vi "TryUpdateDisplacementSample.vi"   [LabVIEW 2016]
uses:
  TelemetryDataTypes.ctl
  TelemetryUpdateModes.ctl
  TelemetryFields.ctl
  <vilib>/rvi/Emulation/niFpgaEmulationIsFPGAContextNoSignature.vi
  <vilib>/rvi/Emulation/niFpgaSctlEmulationGetInTimedLoop.vi
  <vilib>/rvi/errors/niFpgaSetErrorForExecOnDevCompSimple.vi
  <vilib>/rvi/eio/common/nirviEmuReportErrorAndStop.vi
  <vilib>/rvi/DataTransferAndStorage/Container/Common/niFpgaContainerGetUniqueNameForEmu.vi
  <vilib>/rvi/FIFO/Fifo_Resource/nirvififoEmulationSetSize.vi
  <vilib>/rvi/FIFO/Fifo_Resource/nirviFifoEmulationQueueMgr.vi
  <instcachedir>/0/nirviFifoEmulationQueueMgr_E5CAEC123FF24DC58D834DCA3CDAA9B5.lvgen/nirviFifoEmulationQueueMgr_E5CAEC123FF24DC58D834DCA3CDAA9B5_028.vi
  <vilib>/Utility/error.llb/Clear Errors.vi
  <vilib>/rvi/FIFO/Fifo_Resource/nirvififoEmulationCreateLock.vi
  <vilib>/rvi/Emulation/niFpgaProcessEmulError.vi
  <vilib>/rvi/FIFO/Fifo_Resource/nirvififoEmulationObtainLock.vi
  <vilib>/rvi/FIFO/Fifo_Resource/nirvififoEmulationReleaseLock.vi
  <vilib>/rvi/occurrence/nirviWaitOnOccurrenceBase.vi
  <vilib>/rvi/errors/nirviReportUnexpectedCaseInternalError.vi
  <vilib>/rvi/errors/nirviReportUnexpectedCaseInternalError (U32).vi
  <instcachedir>/0/nirviFifoEmulationQueueMgr_E5CAEC123FF24DC58D834DCA3CDAA9B5.lvgen/nirviFifoEmulationQueueMgr_E5CAEC123FF24DC58D834DCA3CDAA9B5_030.vi
  <vilib>/rvi/FIFO/Fifo_Resource/nirvififoEmulationDetermineInputValidOut.vi
  <instcachedir>/0/nirviFifoEmulationQueueMgr_E5CAEC123FF24DC58D834DCA3CDAA9B5.lvgen/nirviFifoEmulationQueueMgr_E5CAEC123FF24DC58D834DCA3CDAA9B5_031.vi
  <vilib>/rvi/Emulation/niFpgaGetClockAttributes.vi
  <vilib>/rvi/Emulation/niFpgaEmulationReportErrorSimple.vi
  <vilib>/rvi/Memory/Memory_Emulation/niFpgaMemoryEmulationCacheClearOnFirstRun.vi
  <vilib>/rvi/Memory/Memory_Emulation/nirvimemoryEmulationManagerCache_MakeExclusive.vi
  <vilib>/rvi/Memory/Memory_Emulation/niFpgaMemoryEmulationValidateCache.vi
  <vilib>/rvi/Memory/Memory_Emulation/nirvimemoryEmulationManagerCache_InsertValue.vi
  <vilib>/rvi/Memory/Memory_Emulation/nirvimemoryEmulationManagerCache_ReleaseExclusive.vi
  <vilib>/rvi/Memory/Memory_Emulation/nirvimemoryEmulationManagerCache_GetValue.vi
  <vilib>/rvi/Memory/Memory_Emulation/nirvimemoryEmulationManagerCache_SetValue.vi
  <vilib>/rvi/Emulation/niFpgaCriticalErrorInLSC.vi
  <instcachedir>/0/nirviFifoEmulationQueueMgr_E5CAEC123FF24DC58D834DCA3CDAA9B5.lvgen/nirviFifoEmulationQueueMgr_E5CAEC123FF24DC58D834DCA3CDAA9B5_004.vi
  <vilib>/rvi/DataTransferAndStorage/Container/XNode/niFpgaContainer.xnode
  <vilib>/rvi/FIFO/Fifo_Resource/nirvififoEmulationRead.vi
  <vilib>/rvi/FIFO/Fifo_Resource/nirvififoEmulationWrite.vi
  <vilib>/rvi/DataTransferAndStorage/Register/Emulation/niFpgaRegisterEmulation.vi
  Displacement/DisplacementErrorCodes.ctl
types:
  T1 = cluster{"Timestamp":u64, "TxBytes":u64, "RxBytes":u64, "TxFrames":u64, "RxFrames":u64, "Sensor1Raw":i32, "Sensor2Raw":i32, "Sensor3Raw":i32, "Sensor4Raw":i32, "Sensor5Raw":i32, "Sensor6Raw":i32, "Sensor7Raw":i32, "Sensor8Raw":i32, "Sensor1Eng":sgl, "Sensor2Eng":sgl, "Sensor3Eng":sgl, "Sensor4Eng":sgl, "Sensor5Eng":sgl, "Sensor6Eng":sgl, "Sensor7Eng":sgl, "Sensor8Eng":sgl, "PositionX":sgl, "PositionY":sgl, "PositionZ":sgl, "RotationX":sgl, "RotationY":sgl, "RotationZ":sgl}
  T2 = typedef "TelemetryFields.ctl" = enum16{"None", "InclinometerTxBytes", "InclinometerRxBytes", "InclinometerTxFrames", "InclinometerRxFrames", "InclinometerErrorTimestamp", "InclinometerErrorCode", "InclinometerSampleTimestamp", "InclinometerRawAngle", "InclinometerZenithAngle", "DisplacementTxBytes", "DisplacementRxBytes", "DisplacementTxFrames", "DisplacementRxFrames", "DisplacementErrorTimestamp", "DisplacementErrorCode", "DisplacementSampleTimestamp", "DisplacementRaw1", "DisplacementRaw2", "DisplacementRaw3", "DisplacementRaw4", "DisplacementRaw5", "DisplacementRaw6", "DisplacementRaw7", "DisplacementRaw8", "DisplacementEng1", "DisplacementEng2", "DisplacementEng3", "DisplacementEng4", "DisplacementEng5", "DisplacementEng6", "DisplacementEng7", "DisplacementEng8", "DisplacementPositionX", "DisplacementPositionY", "DisplacementPositionZ", "DisplacementRotationX", "DisplacementRotationY", "DisplacementRotationZ", "AccelerometerSampleCount", "AccelerometerTimestamp", "AccelerometerRaw1", "AccelerometerRaw2", "AccelerometerRaw3", "AccelerometerRaw4", "AccelerometerRaw5", "AccelerometerRaw6", "AccelerometerRaw7", "AccelerometerRaw8", "AccelerometerEng1", "AccelerometerEng2", "AccelerometerEng3", "AccelerometerEng4", "AccelerometerEng5", "AccelerometerEng6", "AccelerometerEng7", "AccelerometerEng8", "AngularAccelerationX", "AngularAccelerationY", "AngularAccelerationZ"}
  T3 = typedef "TelemetryUpdateModes.ctl" = enum8{"=", "+", "-", "|"}
  T4 = typedef "TelemetryDataTypes.ctl" = enum8{"U8", "U16", "U32", "U64", "I8", "I16", "I32", "I64", "SGL"}
  T5 = typedef "DisplacementErrorCodes.ctl" = enum16{"None", "ResponseUnknownError", "ResponseInvalidError", "ResponseTimeoutError", "SensorIndicatesInvalidCommandError", "SensorIndicatesCommunicationTimeoutError", "SensorIndicatesDataLengthError", "SensorIndicatesNumberOfParametersError", "SensorIndicatesParameterError", "SensorIndicatesCommunicationError", "SensorIndicatesIDNumberError", "SensorIndicatesExpansionLineError", "SensorIndicatesWriteControlError"}
  T6 = typedef "TelemetryUpdateData.ctl" = cluster{"DataType":T4, "Mode":T3, "Field":T2, "Data":u64}
  T7 = typedef "TelemetryUpdateDataSGL.ctl" = cluster{"Mode":T3, "Field":T2, "Data":sgl}
diagram:
  n1 = xnode ("FIFO Method Node")("Timeout"=0) -> ("Element"=w1:T1, "Timed Out?"=w2:bool)  [unwired: 1 in, 1 out]
  n2 = case shown="False" w2 {
    tunnel: w1 -> [w4 _]
    frame False {
      n3 = flat-sequence {
        tunnel: w4 -> [w7]
        tunnel: w4 -> [w13]
        tunnel: w4 -> [w21]
        tunnel: w4 -> [w29]
        tunnel: w4 -> [w37]
        tunnel: w4 -> [w46]
        tunnel: w4 -> [w54]
        tunnel: w4 -> [w62]
        tunnel: w4 -> [w70]
        tunnel: w4 -> [w78]
        tunnel: w4 -> [w86]
        tunnel: w4 -> [w94]
        tunnel: w4 -> [w102]
        tunnel: w4 -> [w110]
        tunnel: w4 -> [w116]
        tunnel: w4 -> [w123]
        tunnel: w4 -> [w130]
        tunnel: w4 -> [w137]
        tunnel: w4 -> [w144]
        tunnel: w4 -> [w151]
        tunnel: w4 -> [w158]
        tunnel: w4 -> [w165]
        tunnel: w4 -> [w172]
        tunnel: w4 -> [w179]
        tunnel: w4 -> [w186]
        tunnel: w4 -> [w193]
        tunnel: w4 -> [w200]
        frame #0 {
          n4 = Unbundle By Name(w7) -> ("Timestamp"=w6:u64)
          n5 = call "GetTelemetryUpdateDataConstant.vi"() -> ("TelemetryUpdateData"=w8:T6)  [unwired: 11 in]
          n6 = Bundle By Name(cluster=w8, "DataType"=TelemetryDataTypes."U64", "Mode"=TelemetryUpdateModes."=", "Field"=TelemetryFields."DisplacementSampleTimestamp" ("TelemetryFields"), "Data"=w6) -> (w11:T6)
          n7 = xnode ("FIFO Method Node")("Element"=w11, "Timeout"=-1) -> ()  [unwired: 1 in, 2 out]
        }
        frame #1 {
          n8 = Unbundle By Name(w13) -> ("TxBytes"=w20:u64)
          n9 = call "GetTelemetryUpdateDataConstant.vi"() -> ("TelemetryUpdateData"=w19:T6)  [unwired: 11 in]
          n10 = Bundle By Name(cluster=w19, "DataType"=TelemetryDataTypes."U64", "Mode"=TelemetryUpdateModes."=", "Field"=TelemetryFields."DisplacementTxBytes", "Data"=w20) -> (w15:T6)
          n11 = xnode ("FIFO Method Node")("Element"=w15, "Timeout"=-1) -> ()  [unwired: 1 in, 2 out]
        }
        frame #2 {
          n12 = Unbundle By Name(w21) -> ("RxBytes"=w22:u64)
          n13 = call "GetTelemetryUpdateDataConstant.vi"() -> ("TelemetryUpdateData"=w23:T6)  [unwired: 11 in]
          n14 = Bundle By Name(cluster=w23, "DataType"=TelemetryDataTypes."U64", "Mode"=TelemetryUpdateModes."=", "Field"=TelemetryFields."DisplacementRxBytes", "Data"=w22) -> (w27:T6)
          n15 = xnode ("FIFO Method Node")("Element"=w27, "Timeout"=-1) -> ()  [unwired: 1 in, 2 out]
        }
        frame #3 {
          n16 = Unbundle By Name(w29) -> ("TxFrames"=w36:u64)
          n17 = call "GetTelemetryUpdateDataConstant.vi"() -> ("TelemetryUpdateData"=w35:T6)  [unwired: 11 in]
          n18 = Bundle By Name(cluster=w35, "DataType"=TelemetryDataTypes."U64", "Mode"=TelemetryUpdateModes."=", "Field"=TelemetryFields."DisplacementTxFrames", "Data"=w36) -> (w31:T6)
          n19 = xnode ("FIFO Method Node")("Element"=w31, "Timeout"=-1) -> ()  [unwired: 1 in, 2 out]
        }
        frame #4 {
          n20 = Unbundle By Name(w37) -> ("RxFrames"=w38:u64)
          n21 = call "GetTelemetryUpdateDataConstant.vi"() -> ("TelemetryUpdateData"=w39:T6)  [unwired: 11 in]
          n22 = Bundle By Name(cluster=w39, "DataType"=TelemetryDataTypes."U64", "Mode"=TelemetryUpdateModes."=", "Field"=TelemetryFields."DisplacementRxFrames", "Data"=w38) -> (w43:T6)
          n23 = xnode ("FIFO Method Node")("Element"=w43, "Timeout"=-1) -> ()  [unwired: 1 in, 2 out]
        }
        frame #5 {
          n24 = Unbundle By Name(w46) -> ("Sensor1Raw"=w52:i32)
          n25 = call "GetTelemetryUpdateDataConstant.vi"() -> ("TelemetryUpdateData"=w51:T6)  [unwired: 11 in]
          n26 = Bundle By Name(cluster=w51, "DataType"=TelemetryDataTypes."I32", "Mode"=TelemetryUpdateModes."=", "Field"=TelemetryFields."DisplacementRaw1" ("TelemetryFields"), "Data"=w52) -> (w48:T6)
          n27 = xnode ("FIFO Method Node")("Element"=w48, "Timeout"=-1) -> ()  [unwired: 1 in, 2 out]
        }
        frame #6 {
          n28 = Unbundle By Name(w54) -> ("Sensor2Raw"=w55:i32)
          n29 = call "GetTelemetryUpdateDataConstant.vi"() -> ("TelemetryUpdateData"=w56:T6)  [unwired: 11 in]
          n30 = Bundle By Name(cluster=w56, "DataType"=TelemetryDataTypes."I32", "Mode"=TelemetryUpdateModes."=", "Field"=TelemetryFields."DisplacementRaw2" ("TelemetryFields"), "Data"=w55) -> (w59:T6)
          n31 = xnode ("FIFO Method Node")("Element"=w59, "Timeout"=-1) -> ()  [unwired: 1 in, 2 out]
        }
        frame #7 {
          n32 = Unbundle By Name(w62) -> ("Sensor3Raw"=w68:i32)
          n33 = call "GetTelemetryUpdateDataConstant.vi"() -> ("TelemetryUpdateData"=w67:T6)  [unwired: 11 in]
          n34 = Bundle By Name(cluster=w67, "DataType"=TelemetryDataTypes."I32", "Mode"=TelemetryUpdateModes."=", "Field"=TelemetryFields."DisplacementRaw3" ("TelemetryFields"), "Data"=w68) -> (w64:T6)
          n35 = xnode ("FIFO Method Node")("Element"=w64, "Timeout"=-1) -> ()  [unwired: 1 in, 2 out]
        }
        frame #8 {
          n36 = Unbundle By Name(w70) -> ("Sensor4Raw"=w71:i32)
          n37 = call "GetTelemetryUpdateDataConstant.vi"() -> ("TelemetryUpdateData"=w72:T6)  [unwired: 11 in]
          n38 = Bundle By Name(cluster=w72, "DataType"=TelemetryDataTypes."I32", "Mode"=TelemetryUpdateModes."=", "Field"=TelemetryFields."DisplacementRaw4" ("TelemetryFields"), "Data"=w71) -> (w75:T6)
          n39 = xnode ("FIFO Method Node")("Element"=w75, "Timeout"=-1) -> ()  [unwired: 1 in, 2 out]
        }
        frame #9 {
          n40 = Unbundle By Name(w78) -> ("Sensor5Raw"=w84:i32)
          n41 = call "GetTelemetryUpdateDataConstant.vi"() -> ("TelemetryUpdateData"=w83:T6)  [unwired: 11 in]
          n42 = Bundle By Name(cluster=w83, "DataType"=TelemetryDataTypes."I32", "Mode"=TelemetryUpdateModes."=", "Field"=TelemetryFields."DisplacementRaw5" ("TelemetryFields"), "Data"=w84) -> (w80:T6)
          n43 = xnode ("FIFO Method Node")("Element"=w80, "Timeout"=-1) -> ()  [unwired: 1 in, 2 out]
        }
        frame #10 {
          n44 = Unbundle By Name(w86) -> ("Sensor6Raw"=w87:i32)
          n45 = call "GetTelemetryUpdateDataConstant.vi"() -> ("TelemetryUpdateData"=w88:T6)  [unwired: 11 in]
          n46 = Bundle By Name(cluster=w88, "DataType"=TelemetryDataTypes."I32", "Mode"=TelemetryUpdateModes."=", "Field"=TelemetryFields."DisplacementRaw6" ("TelemetryFields"), "Data"=w87) -> (w91:T6)
          n47 = xnode ("FIFO Method Node")("Element"=w91, "Timeout"=-1) -> ()  [unwired: 1 in, 2 out]
        }
        frame #11 {
          n48 = Unbundle By Name(w94) -> ("Sensor7Raw"=w100:i32)
          n49 = call "GetTelemetryUpdateDataConstant.vi"() -> ("TelemetryUpdateData"=w99:T6)  [unwired: 11 in]
          n50 = Bundle By Name(cluster=w99, "DataType"=TelemetryDataTypes."I32", "Mode"=TelemetryUpdateModes."=", "Field"=TelemetryFields."DisplacementRaw7" ("TelemetryFields"), "Data"=w100) -> (w96:T6)
          n51 = xnode ("FIFO Method Node")("Element"=w96, "Timeout"=-1) -> ()  [unwired: 1 in, 2 out]
        }
        frame #12 {
          n52 = Unbundle By Name(w102) -> ("Sensor8Raw"=w103:i32)
          n53 = call "GetTelemetryUpdateDataConstant.vi"() -> ("TelemetryUpdateData"=w104:T6)  [unwired: 11 in]
          n54 = Bundle By Name(cluster=w104, "DataType"=TelemetryDataTypes."I32", "Mode"=TelemetryUpdateModes."=", "Field"=TelemetryFields."DisplacementRaw8" ("TelemetryFields"), "Data"=w103) -> (w107:T6)
          n55 = xnode ("FIFO Method Node")("Element"=w107, "Timeout"=-1) -> ()  [unwired: 1 in, 2 out]
        }
        frame #13 {
          n56 = Unbundle By Name(w110) -> ("Sensor1Eng"=w109:sgl)
          n57 = call "GetTelemetryUpdateDataSGLConstant.vi"() -> ("TelemetryUpdateDataSGL"=w115:T7)  [unwired: 11 in]
          n58 = Bundle By Name(cluster=w115, "Mode"=TelemetryUpdateModes."=", "Field"=TelemetryFields."DisplacementEng1", "Data"=w109) -> (w114:T7)
          n59 = xnode ("FIFO Method Node")("Element"=w114, "Timeout"=-1) -> ()  [unwired: 1 in, 2 out]
        }
        frame #14 {
          n60 = Unbundle By Name(w116) -> ("Sensor2Eng"=w122:sgl)
          n61 = call "GetTelemetryUpdateDataSGLConstant.vi"() -> ("TelemetryUpdateDataSGL"=w117:T7)  [unwired: 11 in]
          n62 = Bundle By Name(cluster=w117, "Mode"=TelemetryUpdateModes."=", "Field"=TelemetryFields."DisplacementEng2", "Data"=w122) -> (w118:T7)
          n63 = xnode ("FIFO Method Node")("Element"=w118, "Timeout"=-1) -> ()  [unwired: 1 in, 2 out]
        }
        frame #15 {
          n64 = Unbundle By Name(w123) -> ("Sensor3Eng"=w124:sgl)
          n65 = call "GetTelemetryUpdateDataSGLConstant.vi"() -> ("TelemetryUpdateDataSGL"=w129:T7)  [unwired: 11 in]
          n66 = Bundle By Name(cluster=w129, "Mode"=TelemetryUpdateModes."=", "Field"=TelemetryFields."DisplacementEng3", "Data"=w124) -> (w128:T7)
          n67 = xnode ("FIFO Method Node")("Element"=w128, "Timeout"=-1) -> ()  [unwired: 1 in, 2 out]
        }
        frame #16 {
          n68 = Unbundle By Name(w130) -> ("Sensor4Eng"=w136:sgl)
          n69 = call "GetTelemetryUpdateDataSGLConstant.vi"() -> ("TelemetryUpdateDataSGL"=w131:T7)  [unwired: 11 in]
          n70 = Bundle By Name(cluster=w131, "Mode"=TelemetryUpdateModes."=", "Field"=TelemetryFields."DisplacementEng4", "Data"=w136) -> (w132:T7)
          n71 = xnode ("FIFO Method Node")("Element"=w132, "Timeout"=-1) -> ()  [unwired: 1 in, 2 out]
        }
        frame #17 {
          n72 = Unbundle By Name(w137) -> ("Sensor5Eng"=w138:sgl)
          n73 = call "GetTelemetryUpdateDataSGLConstant.vi"() -> ("TelemetryUpdateDataSGL"=w143:T7)  [unwired: 11 in]
          n74 = Bundle By Name(cluster=w143, "Mode"=TelemetryUpdateModes."=", "Field"=TelemetryFields."DisplacementEng5", "Data"=w138) -> (w142:T7)
          n75 = xnode ("FIFO Method Node")("Element"=w142, "Timeout"=-1) -> ()  [unwired: 1 in, 2 out]
        }
        frame #18 {
          n76 = Unbundle By Name(w144) -> ("Sensor6Eng"=w150:sgl)
          n77 = call "GetTelemetryUpdateDataSGLConstant.vi"() -> ("TelemetryUpdateDataSGL"=w145:T7)  [unwired: 11 in]
          n78 = Bundle By Name(cluster=w145, "Mode"=TelemetryUpdateModes."=", "Field"=TelemetryFields."DisplacementEng6", "Data"=w150) -> (w146:T7)
          n79 = xnode ("FIFO Method Node")("Element"=w146, "Timeout"=-1) -> ()  [unwired: 1 in, 2 out]
        }
        frame #19 {
          n80 = Unbundle By Name(w151) -> ("Sensor7Eng"=w152:sgl)
          n81 = call "GetTelemetryUpdateDataSGLConstant.vi"() -> ("TelemetryUpdateDataSGL"=w157:T7)  [unwired: 11 in]
          n82 = Bundle By Name(cluster=w157, "Mode"=TelemetryUpdateModes."=", "Field"=TelemetryFields."DisplacementEng7", "Data"=w152) -> (w156:T7)
          n83 = xnode ("FIFO Method Node")("Element"=w156, "Timeout"=-1) -> ()  [unwired: 1 in, 2 out]
        }
        frame #20 {
          n84 = Unbundle By Name(w158) -> ("Sensor8Eng"=w164:sgl)
          n85 = call "GetTelemetryUpdateDataSGLConstant.vi"() -> ("TelemetryUpdateDataSGL"=w159:T7)  [unwired: 11 in]
          n86 = Bundle By Name(cluster=w159, "Mode"=TelemetryUpdateModes."=", "Field"=TelemetryFields."DisplacementEng8", "Data"=w164) -> (w160:T7)
          n87 = xnode ("FIFO Method Node")("Element"=w160, "Timeout"=-1) -> ()  [unwired: 1 in, 2 out]
        }
        frame #21 {
          n88 = Unbundle By Name(w165) -> ("PositionX"=w166:sgl)
          n89 = call "GetTelemetryUpdateDataSGLConstant.vi"() -> ("TelemetryUpdateDataSGL"=w171:T7)  [unwired: 11 in]
          n90 = Bundle By Name(cluster=w171, "Mode"=TelemetryUpdateModes."=", "Field"=TelemetryFields."DisplacementPositionX", "Data"=w166) -> (w170:T7)
          n91 = xnode ("FIFO Method Node")("Element"=w170, "Timeout"=-1) -> ()  [unwired: 1 in, 2 out]
        }
        frame #22 {
          n92 = Unbundle By Name(w172) -> ("PositionY"=w178:sgl)
          n93 = call "GetTelemetryUpdateDataSGLConstant.vi"() -> ("TelemetryUpdateDataSGL"=w173:T7)  [unwired: 11 in]
          n94 = Bundle By Name(cluster=w173, "Mode"=TelemetryUpdateModes."=", "Field"=TelemetryFields."DisplacementPositionY", "Data"=w178) -> (w174:T7)
          n95 = xnode ("FIFO Method Node")("Element"=w174, "Timeout"=-1) -> ()  [unwired: 1 in, 2 out]
        }
        frame #23 {
          n96 = Unbundle By Name(w179) -> ("PositionZ"=w180:sgl)
          n97 = call "GetTelemetryUpdateDataSGLConstant.vi"() -> ("TelemetryUpdateDataSGL"=w185:T7)  [unwired: 11 in]
          n98 = Bundle By Name(cluster=w185, "Mode"=TelemetryUpdateModes."=", "Field"=TelemetryFields."DisplacementPositionZ", "Data"=w180) -> (w184:T7)
          n99 = xnode ("FIFO Method Node")("Element"=w184, "Timeout"=-1) -> ()  [unwired: 1 in, 2 out]
        }
        frame #24 {
          n100 = Unbundle By Name(w186) -> ("RotationX"=w192:sgl)
          n101 = call "GetTelemetryUpdateDataSGLConstant.vi"() -> ("TelemetryUpdateDataSGL"=w187:T7)  [unwired: 11 in]
          n102 = Bundle By Name(cluster=w187, "Mode"=TelemetryUpdateModes."=", "Field"=TelemetryFields."DisplacementRotationX", "Data"=w192) -> (w188:T7)
          n103 = xnode ("FIFO Method Node")("Element"=w188, "Timeout"=-1) -> ()  [unwired: 1 in, 2 out]
        }
        frame #25 {
          n104 = Unbundle By Name(w193) -> ("RotationY"=w194:sgl)
          n105 = call "GetTelemetryUpdateDataSGLConstant.vi"() -> ("TelemetryUpdateDataSGL"=w199:T7)  [unwired: 11 in]
          n106 = Bundle By Name(cluster=w199, "Mode"=TelemetryUpdateModes."=", "Field"=TelemetryFields."DisplacementRotationY", "Data"=w194) -> (w198:T7)
          n107 = xnode ("FIFO Method Node")("Element"=w198, "Timeout"=-1) -> ()  [unwired: 1 in, 2 out]
        }
        frame #26 {
          n108 = Unbundle By Name(w200) -> ("RotationZ"=w206:sgl)
          n109 = call "GetTelemetryUpdateDataSGLConstant.vi"() -> ("TelemetryUpdateDataSGL"=w201:T7)  [unwired: 11 in]
          n110 = Bundle By Name(cluster=w201, "Mode"=TelemetryUpdateModes."=", "Field"=TelemetryFields."DisplacementRotationZ", "Data"=w206) -> (w202:T7)
          n111 = xnode ("FIFO Method Node")("Element"=w202, "Timeout"=-1) -> ()  [unwired: 1 in, 2 out]
        }
        frame #27 {
          n112 = disable-structure shown="Disabled" {
            frame Disabled {
              n113 = call "GetTelemetryUpdateDataConstant.vi"() -> ("TelemetryUpdateData"=w207:T6)  [unwired: 11 in]
              n114 = Bundle By Name(cluster=w207, "DataType"=TelemetryDataTypes."U8", "Mode"=TelemetryUpdateModes."=", "Field"=TelemetryFields."DisplacementErrorCode" ("TelemetryFields"), "Data"=DisplacementErrorCodes."None" ("DisplacementErrorCodes")) -> (w209:T6)
              n115 = xnode ("FIFO Method Node")("Element"=w209, "Timeout"=-1) -> ()  [unwired: 1 in, 2 out]
            }
            frame Enabled {
            }
          }
        }
        frame #28 {
          n116 = while {
            stop <- w214 stop-if-true
            n117 = xnode "Register Write"() -> ("Data"=w214:bool)  [unwired: 1 in, 1 out]
          }
        }
        frame #29 {
          n118 = xnode ("FIFO Method Node")("Element"=TRUE, "Timeout"=0) -> ()  [unwired: 1 in, 2 out]
        }
      }
    }
    frame True {
    }
  }
